vi "Set Modbus Handle.vi"(10 "Modbus Master":refnum<class "Modbus Master.lvclass">, 11 "IED in":refnum<class "IED.lvclass">) -> (3 "IED out":refnum<class "IED.lvclass">)   [LabVIEW 2015, in "IED Actor.lvlib" / "IED.lvclass"]
uses:
  IED.lvclass
  <vilib>/Modbus/master/Modbus Master.lvclass
  IED.lvclass/IED.ctl
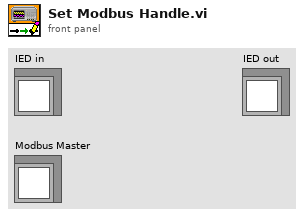
[diagram p1: front panel]
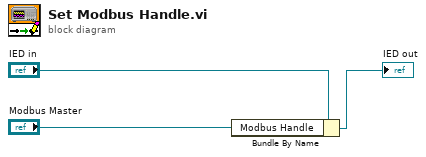
[diagram p0: block diagram]
diagram:
  n1 = Bundle By Name(cluster="IED in", "Modbus Handle"="Modbus Master") -> (→"IED out":refnum<class "IED.lvclass">)
